vi "ReadMerecuryITC_Ethernet.vi"() -> ()   [LabVIEW 2014]
panel:
  out "Reading from the heater controller board (MB0.H1)":string
  in  "error in (no error)":errorcluster
  out "error out":errorcluster
  out "Reading from temperature sensor board (MB1.T1)":string
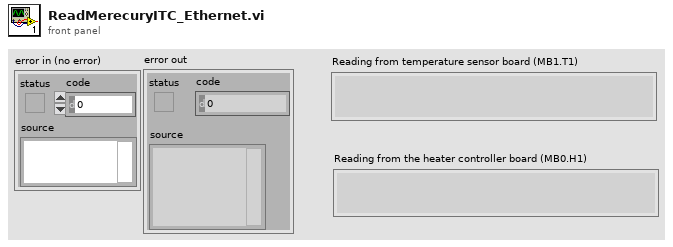
[diagram p1: front panel]
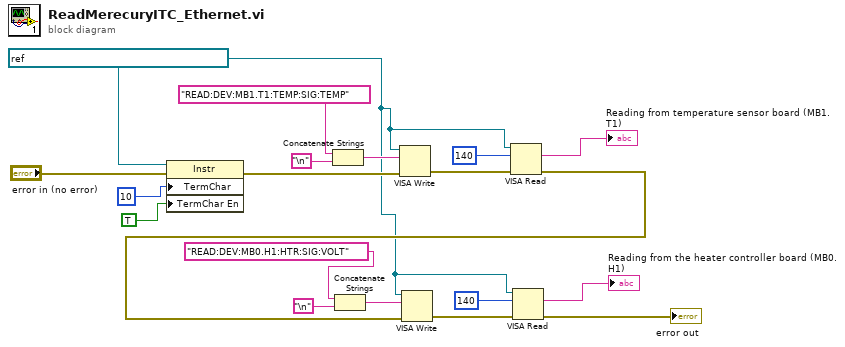
[diagram p0: block diagram]
diagram:
  w1 = refnum<visa-resource-name> "TCPIP0::192.168.128.2::7020::SOCKET" ("VISA resource name")
  n1 = property class="Instr"(reference=w1, error in="error in (no error)", "TermChar"=10, "TermChar En"=TRUE) -> (error out=w3:errorcluster)  [unwired: 1 out]
  n2 = Concatenate Strings("READ:DEV:MB1.T1:TEMP:SIG:TEMP" ("string"), "\n") -> (w16:string)
  n3 = Concatenate Strings("READ:DEV:MB0.H1:HTR:SIG:VOLT" ("string"), "\n") -> (w9:string)
  n4 = VISA Write(VISA resource name=w1, write buffer=w16, error in (no error)=w3) -> (error out=w19:errorcluster)  [unwired: 2 out]
  n5 = VISA Read(VISA resource name=w1, byte count=140, error in (no error)=w19) -> (read buffer=→"Reading from temperature sensor board (MB1.T1)":string, error out=w5:errorcluster)  [unwired: 2 out]
  n6 = VISA Write(VISA resource name=w1, write buffer=w9, error in (no error)=w5) -> (error out=w12:errorcluster)  [unwired: 2 out]
  n7 = VISA Read(VISA resource name=w1, byte count=140, error in (no error)=w12) -> (read buffer=→"Reading from the heater controller board (MB0.H1)":string, error out=→"error out":errorcluster)  [unwired: 2 out]
